vi "PRL BUFFER Cut from Digital 2D Array.vi"(9 "Cut Index":i32, 10 "Signal Index":i32, 11 "Array In":bool[][](array[boolean])) -> (3 "Array Out":bool[](array[boolean]))   [LabVIEW 2013, in "PMU Recorder Light.lvlib"]
uses:
  PMU Recorder Light.lvlib
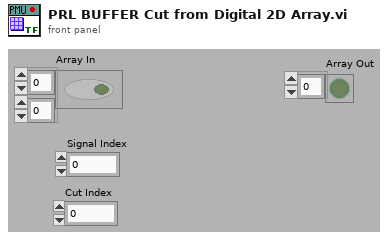
[diagram p1: front panel]
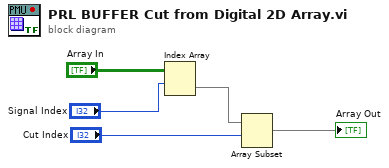
[diagram p0: block diagram]
diagram:
  n1 = Index Array(array="Array In", index (row)="Signal Index") -> (element=w3:bool[])  [unwired: 1 in]
  n2 = Array Subset(array=w3, index="Cut Index") -> (→"Array Out":bool[])  [unwired: 1 in]
